vi "New File Path Create.vi"(11 "Log no":string) -> (0 "에러 출력":errorcluster, 1 "오프셋(바이트)":i64, 3 "바이트 스트림 파일 출력":refnum<file>)   [LabVIEW 2015]
uses:
  <vilib>/Utility/sysdir.llb/System Directory Type.ctl
panel:
  out "경로":path
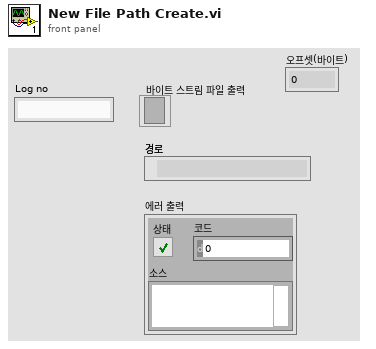
[diagram p1: front panel]
types:
  T1 = enum16{"open", "replace", "create", "open or create", "replace or create", "replace or create with confirmation"}
  T2 = typedef "System Directory Type.ctl" = i32
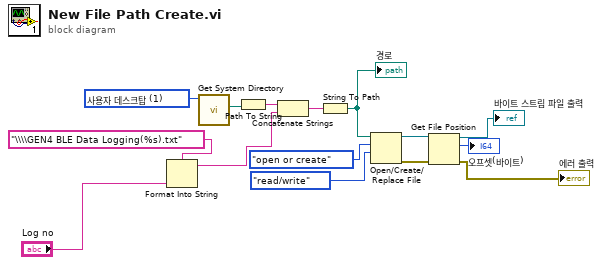
[diagram p0: block diagram]
diagram:
  w6 = T2 1 items=["사용자 홈"=0, "사용자 데스크탑"=1, "사용자 문서"=2, "사용자 어플리케이션 데이터"=3, "사용자 환경"=4, "사용자 임시"=5, "퍼블릭 문서"=6, "퍼블릭 어플리케이션 데이터"=7, "퍼블릭 환경"=8, "퍼블릭 캐시"=13, "시스템 코어 라이브러리"=9, "시스템 설치된 라이브러리"=10, "어플리케이션 파일"=11, "부팅 볼륨 루트"=12] ("system directory type")
  n1 = Format Into String(format string="\\\\GEN4 BLE Data Logging(%s).txt" ("문자열"), "Log no") -> (resulting string=w14:string)  [unwired: 2 in, 1 out]
  n2 = call <vilib>:"Get System Directory.vi"("system directory type"=w6) -> ("system directory"=w7:path)  [unwired: 10 in]
  n3 = Path To String(path=w7) -> (string=w8:string)
  n4 = Concatenate Strings(w8, w14) -> (w9:string)
  n5 = String To Path(string=w9) -> (path=w10:path)
  "경로" <- w10
  n6 = Open/Create/Replace File(file path (use dialog)=w10, operation (0:open)=T1."open or create" ("동작(0:open)"), access (0:read/write)=enum16{"read/write", "read-only", "write-only"}."read/write" ("접근(0:읽기/쓰기)")) -> (refnum out=w4:refnum<file>, error out=w5:errorcluster)  [unwired: 3 in, 1 out]
  n7 = Get File Position(4:w5, 7:w4) -> (0:→"에러 출력":errorcluster, 2:→"오프셋(바이트)":i64, 3:→"바이트 스트림 파일 출력":refnum<file>)
